vi "Save Protocol.vi"(8 "error in (no error)":errorcluster, 11 "Python Protocol in":refnum<class "Python Protocol.lvclass">) -> (0 "error out":errorcluster, 3 "Python Protocol out":refnum<class "Python Protocol.lvclass">)   [LabVIEW 2012, in "Python Protocol Actor.lvlib" / "Python Protocol.lvclass"]
uses:
  Python Protocol.lvclass
  Python Protocol.lvclass/Python Protocol.ctl
  Read Code.vi
  Read Path.vi
  Read Save.vi
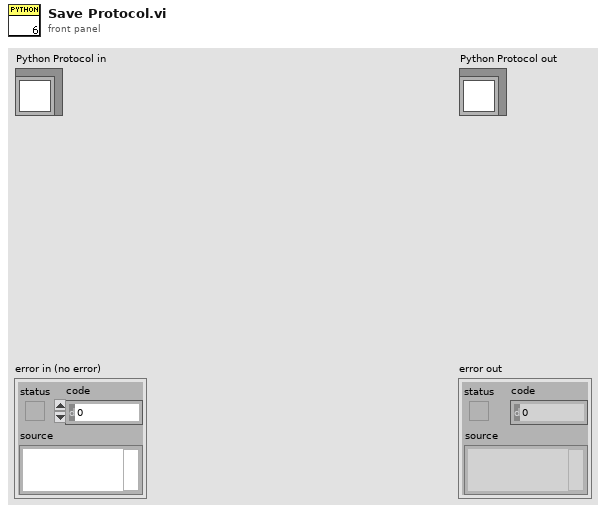
[diagram p1: front panel]
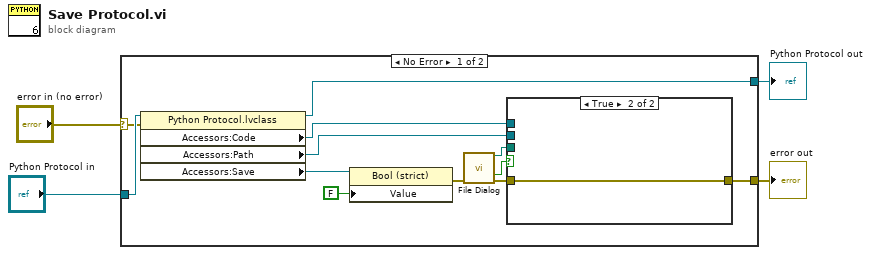
[diagram p0: block diagram]
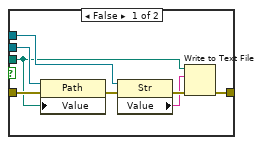
[diagram p2: hidden frame]
diagram:
  n1 = case shown="No Error" "error in (no error)" {
    selector: "error in (no error)" -> [w6 w27]
    tunnel: [w5 w27] -> w3
    tunnel: [w10 w26] -> w1
    tunnel: "Python Protocol in" -> [w11 w26]
    frame No Error {
      n2 = property class="Python Protocol.lvclass"(reference=w11, error in=w6) -> (reference out=w10:refnum<class "Python Protocol.lvclass">, "Accessors:Code"=w9:refnum<vi>, "Accessors:Path"=w8:refnum<vi>, "Accessors:Save"=w7:refnum<vi>)  [unwired: 1 out]
      n3 = property class="Bool (strict)"(reference=w7, "Value"=FALSE) -> (error out=w14:errorcluster)  [unwired: 1 in, 1 out]
      n4 = call "File Dialog"("error in"=w14) -> ("selected path"=w15:path, "cancelled"=w12:bool, "error out"=w16:errorcluster)  [unwired: 11 in, 1 out]
      n5 = case shown="True" w12 {
        tunnel: w9 -> [w24 _]
        tunnel: w16 -> [w23 w25]
        tunnel: w8 -> [w22 _]
        tunnel: w15 -> [w21 _]
        tunnel: [w17 w25] -> w5
        frame False {
          n6 = property class="Path"(reference=w22, error in=w23, "Value"=w21) -> (error out=w20:errorcluster)  [unwired: 1 out]
          n7 = property class="Str"(reference=w24, error in=w20) -> (error out=w19:errorcluster, "Value"=w18:string)  [unwired: 1 out]
          n8 = Write to Text File(file (use dialog)=w21, text=w18, error in=w19) -> (error out=w17:errorcluster)  [unwired: 1 in, 2 out]
        }
        frame True {
        }
      }
    }
    frame Error {
    }
  }
  "error out" <- w3
  "Python Protocol out" <- w1
